vi "Deactivate.vi"(8 "error in (no error)":errorcluster, 11 "BME_DG_Base in":refnum<class "BME_DG_Base.lvclass">) -> (0 "error out":errorcluster, 3 "BME_DG_Base out":refnum<class "BME_DG_Base.lvclass">)   [LabVIEW 2009, in "BME_DG_Base.lvclass"]
uses:
  BME_DG_Base.lvclass
  BME_DG_Base.lvclass/BME_DG_Base.ctl
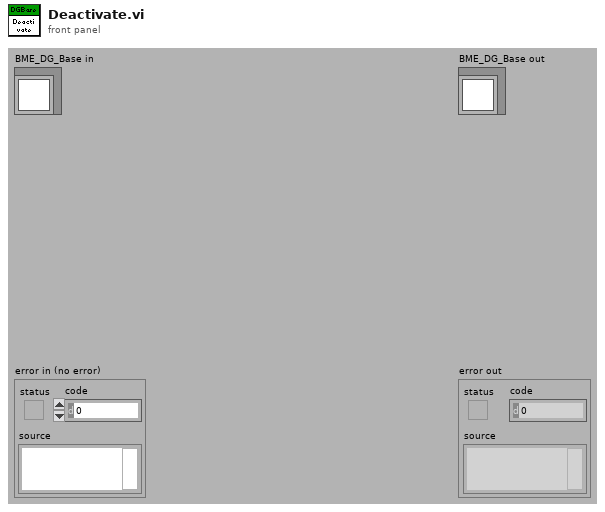
[diagram p1: front panel]
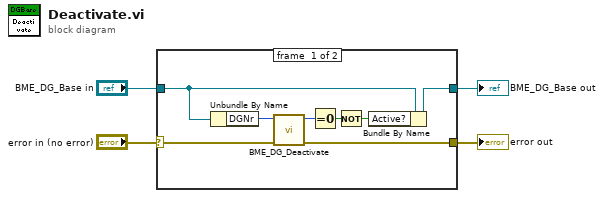
[diagram p0: block diagram]
diagram:
  n1 = case shown="No Error" "error in (no error)" {
    selector: "error in (no error)" -> [w8 w14]
    tunnel: [w7 w14] -> w3
    tunnel: [w11 w13] -> w1
    tunnel: "BME_DG_Base in" -> [w12 w13]
    frame #0 {
      n2 = Unbundle By Name(w12) -> ("DGNr"=w9:i32)
      n3 = call "BME_DG_Deactivate.vi"("error in (no error)"=w8, "DG_Number"=w9) -> ("error out"=w7:errorcluster, "return value"=w6:u32)  [unwired: 8 in]
      n4 = Equal To 0?(x=w6) -> (x = 0?=w10:bool)
      n5 = Not(x=w10) -> (.not. x?=w5:bool)
      n6 = Bundle By Name(cluster=w12, "Active?"=w5) -> (w11:refnum<class "BME_DG_Base.lvclass">)
    }
    frame #1 {
    }
  }
  "error out" <- w3
  "BME_DG_Base out" <- w1
